vi "Example_scatter.vi"() -> ()   [LabVIEW 2015]
uses:
  Controls/lxw_chart_marker_type.ctl
  Controls/lxw_chart_legend_position.ctl
  Controls/lxw_chart_type.ctl
  xlsxwriter.lvlib
panel:
  out "function return 2":string
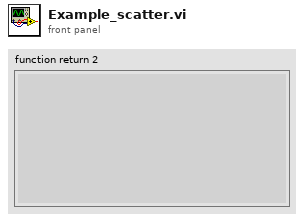
[diagram p1: front panel]
types:
  T1 = enum32{"invalid app kind", "Development System", "Run Time System", "Student Edition", "Embedded LabVIEW", "Evaluation", "Custom"}
  T2 = cluster{"color":u32, "none":u8, "@dummy control@":i8, "@dummy control@":i8, "@dummy control@":i8, "width":sgl, "dash_type":u8, "transparency":u8}
  T3 = cluster{"color":u32, "none":u8, "transparency":u8}
  T4 = typedef "lxw_chart_type.ctl" = u16
  T5 = typedef "lxw_chart_legend_position.ctl" = u8
  T6 = typedef "lxw_chart_marker_type.ctl" = u8
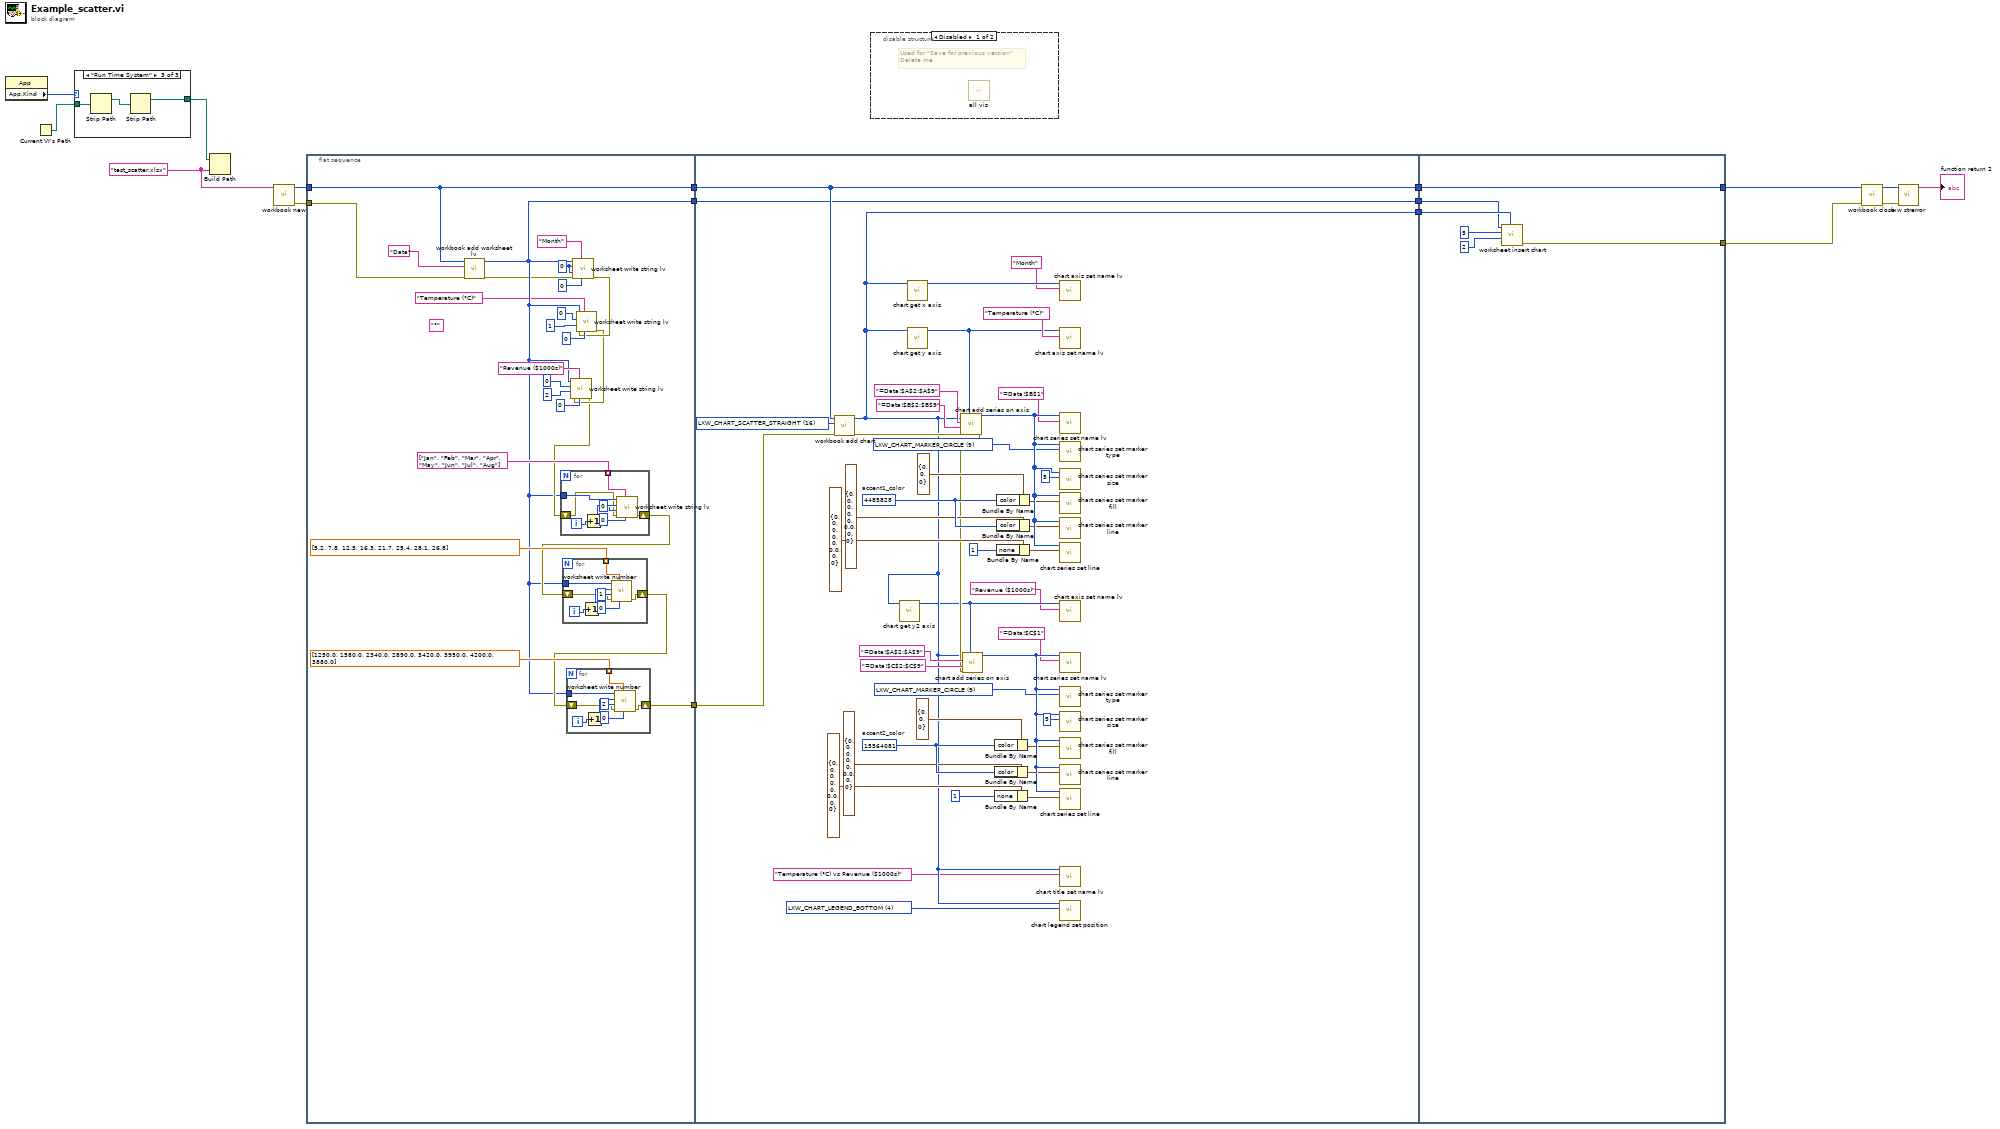
[diagram p0: block diagram]
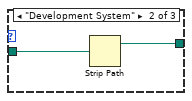
[diagram p4: hidden frame]
diagram:
  w12 = "test_scatter.xlsx" ("filename")
  n1 = property class="App"() -> ("App.Kind"=w16:T1)  [unwired: 2 in, 2 out]
  n2 = Current VI's Path() -> (path=w15:path)
  n3 = case shown="\"Run Time System\"" w16 {
    tunnel: w15 -> [w18 w20 w23]
    tunnel: [w18 w19 w21] -> w14
    frame "invalid app kind", Default {
    }
    frame "Development System" {
      n4 = Strip Path(path=w20) -> (stripped path=w19:path)  [unwired: 1 out]
    }
    frame "Run Time System" {
      n5 = Strip Path(path=w23) -> (stripped path=w22:path)  [unwired: 1 out]
      n6 = Strip Path(path=w22) -> (stripped path=w21:path)  [unwired: 1 out]
    }
  }
  n7 = Build Path(base path=w14, name or relative path=w12) -> ()  [unwired: 1 out]
  n8 = call "workbook new.vi"("filename"=w12) -> ("error out"=w11:errorcluster, "function return"=w17:u32)  [unwired: 9 in]
  n9 = flat-sequence {
    tunnel: w17 -> [w28]
    tunnel: w11 -> [w25]
    tunnel: [w29] -> w10
    tunnel: [w28] -> w3
    tunnel: [w27] -> w1
    tunnel: w10 -> [w94]
    tunnel: [w95] -> w8
    tunnel: [w81] -> w7
    tunnel: w3 -> [w95]
    tunnel: [w78] -> w2
    tunnel: w1 -> [w78]
    tunnel: [w119] -> w9
    tunnel: w8 -> [w120]
    tunnel: w7 -> [w121]
    tunnel: [w120] -> w6
    tunnel: w2 -> [w116]
    frame #0 {
      (unwired) "°"
      w47 = u32 0 ("row")
      n10 = call "workbook add worksheet lv.vi"("error in (no error)"=w25, "sheetname"="Data", "workbook"=w28) -> ("error out"=w24:errorcluster, "function return"=w27:u32)  [unwired: 7 in]
      n11 = call "worksheet write string lv.vi"("format"=u32 0, "string"="Month", "error in (no error)"=w24, "col"=w47, "row"=w47, "worksheet"=w27) -> ("error out"=w34:errorcluster)  [unwired: 4 in, 1 out]
      n12 = call "worksheet write string lv.vi"("format"=u32 0, "string"="Temperature (°C)", "error in (no error)"=w34, "col"=u16 1, "row"=u32 0, "worksheet"=w27) -> ("error out"=w33:errorcluster)  [unwired: 4 in, 1 out]
      n13 = call "worksheet write string lv.vi"("format"=u32 0, "string"="Revenue ($1000s)", "error in (no error)"=w33, "col"=u16 2, "row"=u32 0, "worksheet"=w27) -> ("error out"=w32:errorcluster)  [unwired: 4 in, 1 out]
      n14 = for {
        tunnel: w27 -> [w72]
        tunnel: string[] ["Jan", "Feb", "Mar", "Apr", "May", "Jun", "Jul", "Aug"] -> [w67] mode=indexing
        shift-right: [w65] -> w31
        shift-left: w32 -> [w66]
        i -> [w71]
        n15 = Increment(x=w71) -> (x+1=w70:i32)
        n16 = call "worksheet write string lv.vi"("format"=u32 0, "string"=w67, "error in (no error)"=w66, "col"=u16 0, "row"=w70, "worksheet"=w72) -> ("error out"=w65:errorcluster)  [unwired: 4 in, 1 out]
      }
      n17 = for {
        tunnel: w27 -> [w64]
        tunnel: dbl[] [5.2, 7.8, 12.5, 16.3, 21.7, 25.4, 28.1, 26.8] -> [w63] mode=indexing
        shift-right: [w57] -> w30
        shift-left: w31 -> [w58]
        i -> [w62]
        n18 = Increment(x=w62) -> (x+1=w61:i32)
        n19 = call "worksheet write number.vi"("format"=u32 0, "number"=w63, "error in (no error)"=w58, "col"=u16 1, "row"=w61, "worksheet"=w64) -> ("error out"=w57:errorcluster)  [unwired: 4 in, 1 out]
      }
      n20 = for {
        tunnel: w27 -> [w56]
        tunnel: dbl[] [1250.0, 1580.0, 2340.0, 2890.0, 3420.0, 3950.0, 4200.0, 3880.0] -> [w55] mode=indexing
        shift-right: [w49] -> w29
        shift-left: w30 -> [w50]
        i -> [w54]
        n21 = Increment(x=w54) -> (x+1=w53:i32)
        n22 = call "worksheet write number.vi"("format"=u32 0, "number"=w55, "error in (no error)"=w50, "col"=u16 2, "row"=w53, "worksheet"=w56) -> ("error out"=w49:errorcluster)  [unwired: 4 in, 1 out]
      }
    }
    frame #1 {
      w73 = T4 16 items=["LXW_CHART_NONE", "LXW_CHART_AREA", "LXW_CHART_AREA_STACKED", "LXW_CHART_AREA_STACKED_PERCENT", "LXW_CHART_BAR", "LXW_CHART_BAR_STACKED", "LXW_CHART_BAR_STACKED_PERCENT", "LXW_CHART_COLUMN", "LXW_CHART_COLUMN_STACKED", "LXW_CHART_COLUMN_STACKED_PERCENT", "LXW_CHART_DOUGHNUT", "LXW_CHART_LINE", "LXW_CHART_LINE_STACKED", "LXW_CHART_LINE_STACKED_PERCENT", "LXW_CHART_PIE", "LXW_CHART_SCATTER", "LXW_CHART_SCATTER_STRAIGHT", "LXW_CHART_SCATTER_STRAIGHT_WITH_MARKERS", "LXW_CHART_SCATTER_SMOOTH", "LXW_CHART_SCATTER_SMOOTH_WITH_MARKERS", "LXW_CHART_RADAR", "LXW_CHART_RADAR_WITH_MARKERS", "LXW_CHART_RADAR_FILLED"] ("Ring")
      w79 = T5 4 items=["LXW_CHART_LEGEND_NONE", "LXW_CHART_LEGEND_RIGHT", "LXW_CHART_LEGEND_LEFT", "LXW_CHART_LEGEND_TOP", "LXW_CHART_LEGEND_BOTTOM", "LXW_CHART_LEGEND_TOP_RIGHT", "LXW_CHART_LEGEND_OVERLAY_RIGHT", "LXW_CHART_LEGEND_OVERLAY_LEFT"] ("position")
      w102 = T6 9 items=["LXW_CHART_MARKER_AUTOMATIC", "LXW_CHART_MARKER_NONE", "LXW_CHART_MARKER_SQUARE", "LXW_CHART_MARKER_DIAMOND", "LXW_CHART_MARKER_TRIANGLE", "LXW_CHART_MARKER_X", "LXW_CHART_MARKER_STAR", "LXW_CHART_MARKER_SHORT_DASH", "LXW_CHART_MARKER_LONG_DASH", "LXW_CHART_MARKER_CIRCLE", "LXW_CHART_MARKER_PLUS"] ("type")
      w101 = T6 9 items=["LXW_CHART_MARKER_AUTOMATIC", "LXW_CHART_MARKER_NONE", "LXW_CHART_MARKER_SQUARE", "LXW_CHART_MARKER_DIAMOND", "LXW_CHART_MARKER_TRIANGLE", "LXW_CHART_MARKER_X", "LXW_CHART_MARKER_STAR", "LXW_CHART_MARKER_SHORT_DASH", "LXW_CHART_MARKER_LONG_DASH", "LXW_CHART_MARKER_CIRCLE", "LXW_CHART_MARKER_PLUS"] ("type")
      w112 = u32 15564081  # accent2_color
      w106 = u32 4485828  # accent1_color
      n23 = call "workbook add chart.vi"("error in (no error)"=w94, "Ring"=w73, "workbook"=w95) -> ("error out"=w93:errorcluster, "function return"=w81:u32)  [unwired: 7 in]
      n24 = call "chart get y2 axis.vi"("chart"=w81) -> ("function return"=w75:u32)  [unwired: 9 in, 1 out]
      n25 = call "chart get x axis.vi"("chart"=w81) -> ("function return"=w83:u32)  [unwired: 9 in, 1 out]
      n26 = call "chart get y axis.vi"("chart"=w81) -> ("function return"=w76:u32)  [unwired: 9 in, 1 out]
      n27 = call "chart add series on axis.vi"("y_axis"=w76, "error in (no error)"=w93, "values"="=Data!$B$2:$B$9", "categories"="=Data!$A$2:$A$9", "chart"=w81) -> ("error out"=w92:errorcluster, "function return"=w115:u32)  [unwired: 5 in]
      n28 = call "chart add series on axis.vi"("y_axis"=w75, "error in (no error)"=w92, "values"="=Data!$C$2:$C$9", "categories"="=Data!$A$2:$A$9", "chart"=w81) -> ("function return"=w113:u32)  [unwired: 5 in, 1 out]
      n29 = Bundle By Name(cluster=T3 {"color"=0, "none"=0, "transparency"=0} ("fill"), "color"=w112) -> (w86:T3)
      n30 = Bundle By Name(cluster=T2 {"color"=0, "none"=0, "@dummy control@"=0, "@dummy control@"=0, "@dummy control@"=0, "width"=0.0, "dash_type"=0, "transparency"=0} ("line"), "color"=w112) -> (w84:T2)
      n31 = Bundle By Name(cluster=T2 {"color"=0, "none"=0, "@dummy control@"=0, "@dummy control@"=0, "@dummy control@"=0, "width"=0.0, "dash_type"=0, "transparency"=0} ("line"), "none"=u8 1) -> (w85:T2)
      n32 = Bundle By Name(cluster=T3 {"color"=0, "none"=0, "transparency"=0} ("fill"), "color"=w106) -> (w90:T3)
      n33 = Bundle By Name(cluster=T2 {"color"=0, "none"=0, "@dummy control@"=0, "@dummy control@"=0, "@dummy control@"=0, "width"=0.0, "dash_type"=0, "transparency"=0} ("line"), "color"=w106) -> (w89:T2)
      n34 = Bundle By Name(cluster=T2 {"color"=0, "none"=0, "@dummy control@"=0, "@dummy control@"=0, "@dummy control@"=0, "width"=0.0, "dash_type"=0, "transparency"=0} ("line"), "none"=u8 1) -> (w88:T2)
      n35 = call "chart axis set name lv.vi"("name"="Month", "axis"=w83) -> ()  [unwired: 9 in, 1 out]
      n36 = call "chart axis set name lv.vi"("name"="Temperature (°C)", "axis"=w76) -> ()  [unwired: 9 in, 1 out]
      n37 = call "chart series set name lv.vi"("name"="=Data!$B$1", "series"=w115) -> ()  [unwired: 9 in, 1 out]
      n38 = call "chart series set marker type.vi"("type"=w101, "series"=w115) -> ()  [unwired: 9 in, 1 out]
      n39 = call "chart series set marker size.vi"("size"=u8 5, "series"=w115) -> ()  [unwired: 9 in, 1 out]
      n40 = call "chart series set marker fill.vi"("fill"=w90, "series"=w115) -> ()  [unwired: 8 in, 2 out]
      n41 = call "chart series set marker line.vi"("line"=w89, "series"=w115) -> ()  [unwired: 8 in, 2 out]
      n42 = call "chart series set line.vi"("line"=w88, "series"=w115) -> ()  [unwired: 8 in, 2 out]
      n43 = call "chart axis set name lv.vi"("name"="Revenue ($1000s)", "axis"=w75) -> ()  [unwired: 9 in, 1 out]
      n44 = call "chart series set name lv.vi"("name"="=Data!$C$1", "series"=w113) -> ()  [unwired: 9 in, 1 out]
      n45 = call "chart series set marker type.vi"("type"=w102, "series"=w113) -> ()  [unwired: 9 in, 1 out]
      n46 = call "chart series set marker size.vi"("size"=u8 5, "series"=w113) -> ()  [unwired: 9 in, 1 out]
      n47 = call "chart series set marker fill.vi"("fill"=w86, "series"=w113) -> ()  [unwired: 8 in, 2 out]
      n48 = call "chart series set marker line.vi"("line"=w84, "series"=w113) -> ()  [unwired: 8 in, 2 out]
      n49 = call "chart series set line.vi"("line"=w85, "series"=w113) -> ()  [unwired: 8 in, 2 out]
      n50 = call "chart title set name lv.vi"("name"="Temperature (°C) vs Revenue ($1000s)", "chart"=w81) -> ()  [unwired: 9 in, 1 out]
      n51 = call "chart legend set position.vi"("position"=w79, "chart"=w81) -> ()  [unwired: 9 in, 1 out]
    }
    frame #2 {
      n52 = call "worksheet insert chart.vi"("chart"=w121, "col"=u16 2, "row"=u32 5, "worksheet"=w116) -> ("error out"=w119:errorcluster)  [unwired: 6 in, 1 out]
    }
  }
  n53 = disable-structure shown="Disabled" {
    frame Disabled {
      # "Used for \"Save for previous version\"\nDelete me"
      n54 = call "all vis.vi"() -> ()  [unwired: 12 in]
    }
    frame Enabled {
    }
  }
  n55 = call "workbook close.vi"("error in (no error)"=w9, "workbook"=w6) -> ("error out"=w5:errorcluster, "function return"=w13:u32)  [unwired: 8 in]
  n56 = call "lxw strerror.vi"("error in (no error)"=w5, "error_num"=w13) -> ("function return"=→"function return 2":string)  [unwired: 8 in, 1 out]
